vi "cluster.vi"() -> ()   [LabVIEW 2009]
uses:
  <vilib>/NXT/Block Support/NXT_OutputPort.ctl
panel:
  out "Cluster":cluster{"Degrees out":i32, "Degrees out":i32}
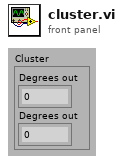
[diagram p1: front panel]
types:
  T1 = typedef "NXT_OutputPort.ctl" = u8
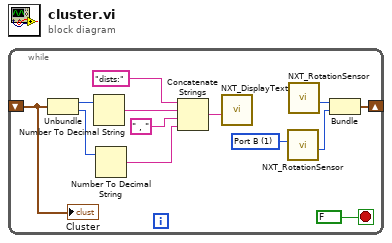
[diagram p0: block diagram]
diagram:
  n1 = while {
    shift-right: [w13] -> _
    shift-left: _ -> [w12]
    stop <- FALSE stop-if-true
    w5 = T1 1 items=["Port A", "Port B", "Port C"] ("Output (Port A)")
    n2 = Unbundle(w12) -> ("Degrees out"=w10:i32, "Degrees out"=w3:i32)
    n3 = Number To Decimal String(number=w10) -> (decimal integer string=w9:string)  [unwired: 1 in]
    n4 = Number To Decimal String(number=w3) -> (decimal integer string=w1:string)  [unwired: 1 in]
    n5 = Concatenate Strings("dists:" ("string"), w9, " , " ("string"), w1) -> (w7:string)
    n6 = call <vilib>:"NXT_DisplayText.vi"("Text"=w7) -> ()  [unwired: 10 in, 1 out]
    n7 = call <vilib>:"NXT_RotationSensor.vi"("Output (Port A)"=w5) -> ("Degrees out"=w4:i32)  [unwired: 7 in, 3 out]
    n8 = call <vilib>:"NXT_RotationSensor.vi"() -> ("Degrees out"=w11:i32)  [unwired: 8 in, 3 out]
    n9 = Bundle("Degrees out"=w11, "Degrees out"=w4) -> (w13:cluster{"Degrees out":i32, "Degrees out":i32})  [unwired: 1 in]
    "Cluster" <- w12
  }
